vi "manual_mode.vi"(0 "Speed":u8, 1 "Turn":i16(knob)=20 min=-30 max=30 step=1 scale=-30.0..30.0, 2 "Lift":i16(knob)=20 min=-50 max=80 step=1 scale=-50.0..80.0, 3 "POWER":bool, 5 "LEG1":bool, 7 "LEG2":bool, 9 "LEG3":bool, 11 "LEG4":bool, 12 "LEG5":bool, 13 "LEG6":bool) -> (4 "String":string)   [LabVIEW 2012]
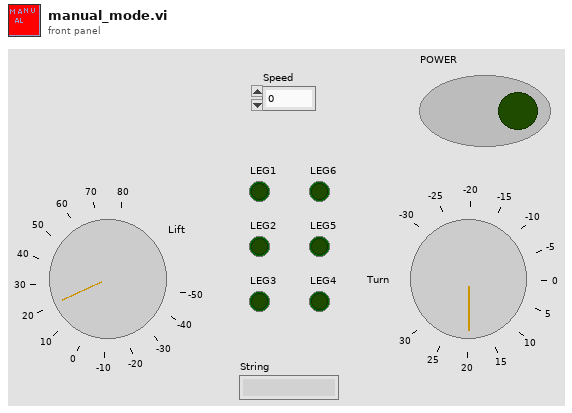
[diagram p1: front panel]
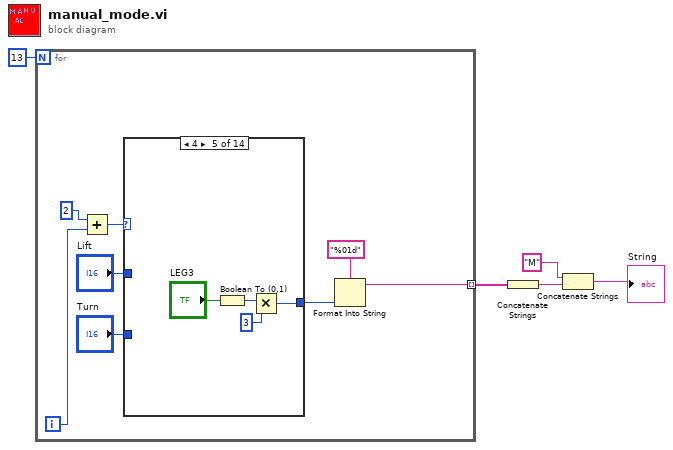
[diagram p0: block diagram]
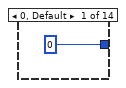
[diagram p2: hidden frame]
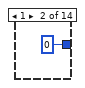
[diagram p3: hidden frame]
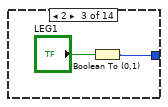
[diagram p4: hidden frame]
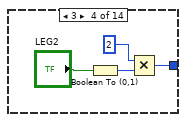
[diagram p5: hidden frame]
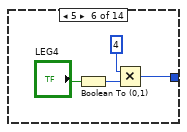
[diagram p6: hidden frame]
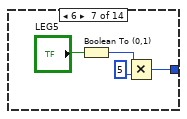
[diagram p7: hidden frame]
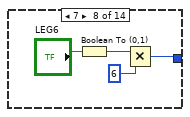
[diagram p8: hidden frame]
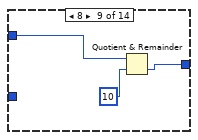
[diagram p9: hidden frame]
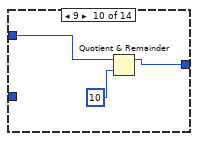
[diagram p10: hidden frame]
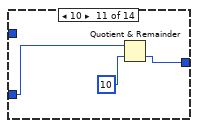
[diagram p11: hidden frame]
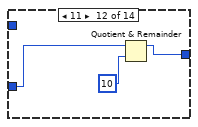
[diagram p12: hidden frame]
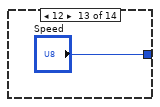
[diagram p13: hidden frame]
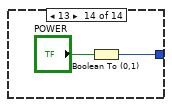
[diagram p14: hidden frame]
diagram:
  n1 = for {
    N: 13 -> [_]
    tunnel: [w7] -> w4 mode=indexing
    i -> [w8]
    n2 = Add(x=2, y=w8) -> (x+y=w9:i32)
    n3 = case shown="4" w9 {
      tunnel: [i16 0 ("Speed") i16 0 ("Speed") w16 w19 w22 w27 w30 w34 w39 w42 w44 w47 "Speed" w51] -> w12
      tunnel: "Lift" -> [_ _ _ _ _ _ _ _ w38 w41 _ _ _ _]
      tunnel: "Turn" -> [_ _ _ _ _ _ _ _ _ _ w45 w48 _ _]
      frame 0, Default {
      }
      frame 1 {
      }
      frame 2 {
        n4 = Boolean To (0,1)(Boolean="LEG1") -> (0, 1=w16:i16)
      }
      frame 3 {
        n5 = Boolean To (0,1)(Boolean="LEG2") -> (0, 1=w20:i16)
        n6 = Multiply(x=i16 2 ("y"), y=w20) -> (x*y=w19:i16)
      }
      frame 4 {
        n7 = Boolean To (0,1)(Boolean="LEG3") -> (0, 1=w23:i16)
        n8 = Multiply(x=w23, y=i16 3) -> (x*y=w22:i16)
      }
      frame 5 {
        n9 = Boolean To (0,1)(Boolean="LEG4") -> (0, 1=w29:i16)
        n10 = Multiply(x=i16 4, y=w29) -> (x*y=w27:i16)
      }
      frame 6 {
        n11 = Boolean To (0,1)(Boolean="LEG5") -> (0, 1=w32:i16)
        n12 = Multiply(x=w32, y=i16 5) -> (x*y=w30:i16)
      }
      frame 7 {
        n13 = Boolean To (0,1)(Boolean="LEG6") -> (0, 1=w36:i16)
        n14 = Multiply(x=w36, y=i16 6) -> (x*y=w34:i16)
      }
      frame 8 {
        n15 = Quotient & Remainder(x=w38, y=i16 10) -> (floor(x/y)=w39:i16)  [unwired: 1 out]
      }
      frame 9 {
        n16 = Quotient & Remainder(x=w41, y=i16 10) -> (x-y*floor(x/y)=w42:i16)  [unwired: 1 out]
      }
      frame 10 {
        n17 = Quotient & Remainder(x=w45, y=i16 10) -> (floor(x/y)=w44:i16)  [unwired: 1 out]
      }
      frame 11 {
        n18 = Quotient & Remainder(x=w48, y=i16 10) -> (x-y*floor(x/y)=w47:i16)  [unwired: 1 out]
      }
      frame 12 {
      }
      frame 13 {
        n19 = Boolean To (0,1)(Boolean="POWER") -> (0, 1=w51:i16)
      }
    }
    n20 = Format Into String(format string="%01d", w12) -> (resulting string=w7:string)  [unwired: 2 in, 1 out]
  }
  n21 = Concatenate Strings(w4) -> (w3:string)
  n22 = Concatenate Strings("M" ("string"), w3) -> (→"String":string)
